vi "readFromXML.vi"(8 "error in (no error)":errorcluster, 10 "XML in":string="<Rotator>\n<rotPA>1.1232</rotPA>\n<rotatorFrame>FK5</rotatorFrame>\n</Rotator>", 11 "Rotator in":refnum<class "Rotator.lvclass">) -> (0 "error out":errorcluster, 3 "Rotator out":refnum<class "Rotator.lvclass">)   [LabVIEW 2022 SP3, in "TCSDataDefinitions.lvlib" / "TCSCommand.lvlib" / "TargetConfiguration.lvlib" / "Rotator.lvclass"]
uses:
  Rotator.lvclass
  RotatorCommands/Enumerations/RotatorFrameValues.ctl
  <userlib>/Common/UnitsAndXML/FlattenItemWithUnitToXML/FlattenPlaneAngleToXML/PlaneAngleUnit.ctl
  Rotator.lvclass/Rotator.ctl
  <userlib>/Common/UnitsAndXML/UnitsAndXML.lvlib
  <userlib>/Common/XML/XMLParser/XMLParser.lvclass
  TCSCommand.lvlib
panel:
  out "rotatorFramVales":T1=enum."Fixed"
  out "planeAngle":dbl[unit]=0.01960353815840031
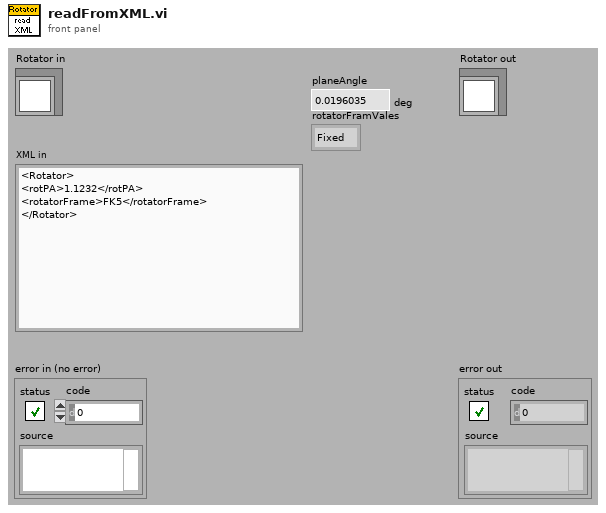
[diagram p1: front panel]
types:
  T1 = typedef "TCSDataDefinitions.lvlib/TCSCommand.lvlib/RotatorFrameValues.ctl" = enum16{"Target", "Fixed"}
  T2 = typedef "UnitsAndXML.lvlib/PlaneAngleUnit.ctl" = enum16{"rad", "deg", "'", "\""}
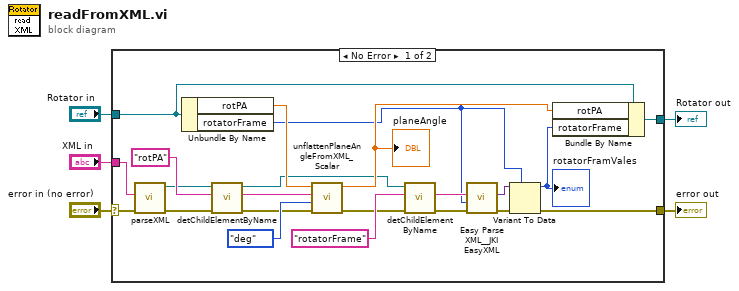
[diagram p0: block diagram]
diagram:
  n1 = case shown="No Error" "error in (no error)" {
    selector: "error in (no error)" -> [w22 w29]
    tunnel: [w8 w29] -> w4
    tunnel: [w23 w28] -> w2
    tunnel: "Rotator in" -> [w21 w28]
    tunnel: "XML in" -> [w27 _]
    frame No Error {
      n2 = call <userlib>:"parseXML.vi"("error in (no error)"=w22, "XMLString in"=w27) -> ("error out"=w26:errorcluster, "Element out"=w7:refnum<class "XMLParser.lvclass">)  [unwired: 8 in]
      n3 = Unbundle By Name(w21) -> ("rotPA"=w20:dbl[unit], "rotatorFrame"=w10:T1)
      n4 = call <userlib>:"detChildElementByName.vi"("error in (no error)"=w26, "childName"="rotPA" ("ChildName"), "Element in"=w7) -> ("error out"=w17:errorcluster, "childXML"=w19:string, "Element out"=w6:refnum<class "XMLParser.lvclass">)  [unwired: 5 in, 1 out]
      n5 = call <userlib>:"unflattenPlaneAngleFromXML_Scalar.vi"("error in (no error)"=w17, "planeAngleUnitInXML"=PlaneAngleUnit."deg", "xmlString"=w19, "planeAngleForType"=w20) -> ("error out"=w16:errorcluster, "planeAngle"=w15:dbl[unit])  [unwired: 6 in]
      "planeAngle" <- w15
      n6 = call <userlib>:"detChildElementByName.vi"("error in (no error)"=w16, "childName"="rotatorFrame" ("ChildName"), "Element in"=w6) -> ("error out"=w13:errorcluster, "childXML"=w14:string)  [unwired: 5 in, 2 out]
      n7 = call <vilib>:"Easy Parse XML__JKI EasyXML.vi"("error in (no error)"=w13, "LabVIEW Data (Type)"=w10, "XML String"=w14) -> ("error out"=w11:errorcluster, "LabVIEW Data"=w12:variant)  [unwired: 7 in]
      n8 = Variant To Data(error in=w11, type=w10, Variant=w12) -> (data=w9:T1, error out=w8:errorcluster)
      "rotatorFramVales" <- w9
      n9 = Bundle By Name(cluster=w21, "rotPA"=w15, "rotatorFrame"=w9) -> (w23:refnum<class "Rotator.lvclass">)
    }
    frame Error {
    }
  }
  "error out" <- w4
  "Rotator out" <- w2
